vi "rad_s to ticks_s.vi"(8 "error in (no error)":errorcluster, 10 "velocity (rad/s)":dbl, 11 "KUKA youBot arm motor_EtherCAT in":refnum<class "NI_Robotics_KUKA youBot Arm Motor_EtherCAT.lvclass">) -> (0 "error out":errorcluster, 2 "ticks/s":i32=1, 3 "KUKA youBot arm motor_EtherCAT out":refnum<class "NI_Robotics_KUKA youBot Arm Motor_EtherCAT.lvclass">)   [LabVIEW 2017, in "NI_Robotics_KUKA youBot Host.lvlib" / "NI_Robotics_KUKA youBot Arm Motor_EtherCAT.lvclass"]
uses:
  <vilib>/robotics/KUKA youBot/Motor/Arm Motor EtherCAT/NI_Robotics_KUKA youBot Arm Motor_EtherCAT.lvclass
  <vilib>/robotics/KUKA youBot/Motor/Arm Motor EtherCAT/NI_Robotics_KUKA youBot Arm Motor_EtherCAT.lvclass/NI_Robotics_KUKA youBot Arm Motor_EtherCAT.ctl
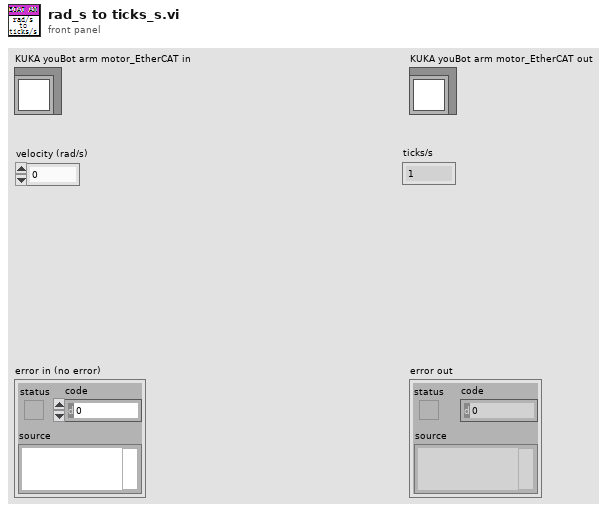
[diagram p1: front panel]
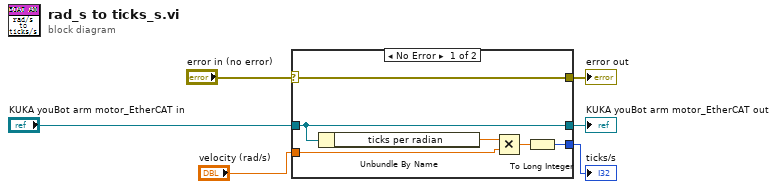
[diagram p0: block diagram]
diagram:
  n1 = case shown="No Error" "error in (no error)" {
    selector: "error in (no error)" -> [w12 w14]
    tunnel: [w12 w14] -> w5
    tunnel: [w11 w13] -> w3
    tunnel: "KUKA youBot arm motor_EtherCAT in" -> [w11 w13]
    tunnel: "velocity (rad/s)" -> [w9 _]
    tunnel: [w7 _] -> w1
    frame No Error {
      n2 = Unbundle By Name(w11) -> ("ticks per radian"=w10:dbl)
      n3 = Multiply(x=w10, y=w9) -> (x*y=w8:dbl)
      n4 = To Long Integer(number=w8) -> (32bit integer=w7:i32)
    }
    frame Error {
    }
  }
  "error out" <- w5
  "KUKA youBot arm motor_EtherCAT out" <- w3
  "ticks/s" <- w1
